vi "DEBUG Query Class.vi"() -> ()   [LabVIEW 2013]
panel:
  in  "Stop Button":bool
  out "Types":string[](array[string])
  out "Type Strings":string[](array[string])
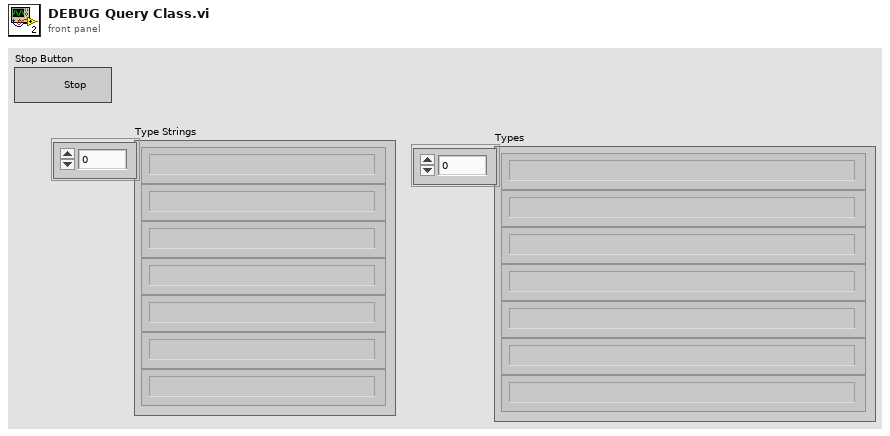
[diagram p1: front panel]
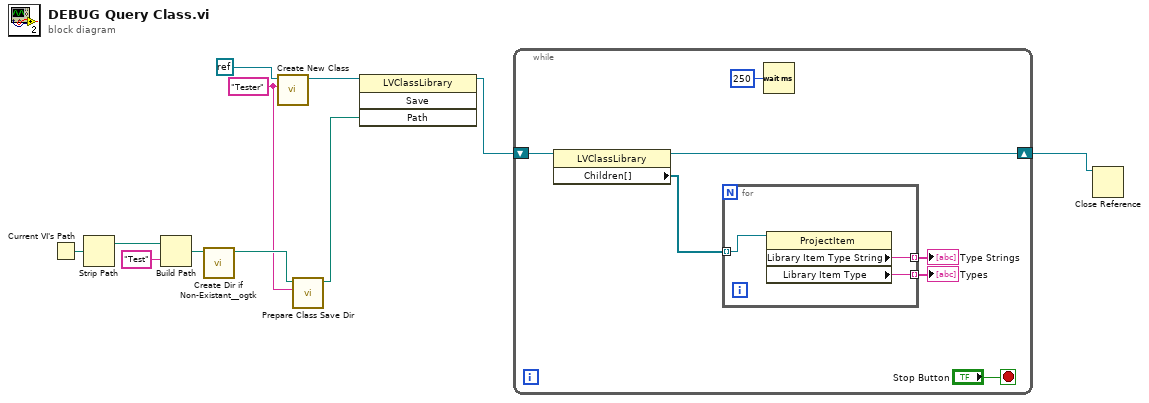
[diagram p0: block diagram]
diagram:
  w3 = "Tester" ("Class Name")
  n1 = Current VI's Path() -> (path=w7:path)
  n2 = Strip Path(path=w7) -> (stripped path=w6:path)  [unwired: 1 out]
  n3 = Build Path(base path=w6, name or relative path="Test") -> (appended path=w5:path)
  n4 = call <userlib>:"Create Dir if Non-Existant__ogtk.vi"("Directory Path"=w5) -> ("dup Directory Path"=w4:path)  [unwired: 8 in, 2 out]
  n5 = call "Create New Class.vi"("Class Name"=w3, "Base Class"=refnum<k0> refnum) -> ("New Class"=w10:refnum<vi>)  [unwired: 8 in, 1 out]
  n6 = call "Prepare Class Save Dir.vi"("Class Name"=w3, "Root Save Dir"=w4) -> ("Class Save Dir"=w2:path)  [unwired: 9 in]
  n7 = invoke class="LVClassLibrary" method="Save"(reference=w10, "Path"=w2) -> (reference out=w9:refnum<vi>)  [unwired: 2 in, 3 out]
  n8 = while {
    shift-right: [w16] -> w1
    shift-left: w9 -> [w17]
    stop <- "Stop Button" stop-if-true
    n9 = property class="LVClassLibrary"(reference=w17) -> (reference out=w16:refnum<vi>, "Children[]"=w15:refnum<vi>[])  [unwired: 1 in, 1 out]
    n10 = for {
      tunnel: w15 -> [w21] mode=indexing
      tunnel: [w20] -> w14 mode=indexing
      tunnel: [w19] -> w13 mode=indexing
      n11 = property class="ProjectItem"(reference=w21) -> ("Library Item Type String"=w20:string, "Library Item Type"=w19:string)  [unwired: 1 in, 2 out]
    }
    "Type Strings" <- w14
    "Types" <- w13
    n12 = Wait (ms)(milliseconds to wait=u32 250) -> ()  [unwired: 1 out]
  }
  n13 = Close Reference(reference=w1) -> ()  [unwired: 1 in, 1 out]
